vi "PlayinwithRIGOL.vi"() -> ()   [LabVIEW 2009]
panel:
  in  "Wait Duration (us)":dbl
  in  "Pulse Duration (us)":dbl
  in  "Ncycles":u16
  in  "Frequency (MHz)":dbl
  in  "Amplitude (Vpp)":dbl
  in  "Phase (degrees 0-360)":dbl
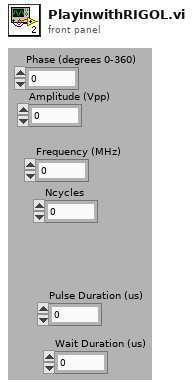
[diagram p1: front panel]
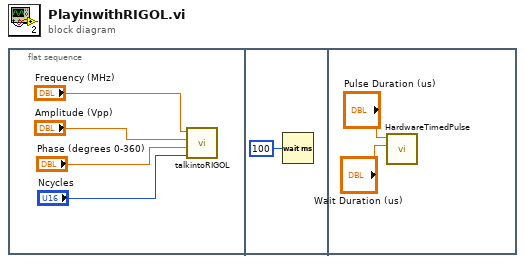
[diagram p0: block diagram]
diagram:
  n1 = flat-sequence {
    frame #0 {
      n2 = call "talkintoRIGOL.vi"("Ncycles"="Ncycles", "Phase (degrees 0-360)"="Phase (degrees 0-360)", "Amplitude (Vpp)"="Amplitude (Vpp)", "Frequency (MHz)"="Frequency (MHz)") -> ()  [unwired: 8 in]
    }
    frame #1 {
      n3 = Wait (ms)(milliseconds to wait=u32 100) -> ()  [unwired: 1 out]
    }
    frame #2 {
      n4 = call "HardwareTimedPulse.vi"("Wait Duration (us)"="Wait Duration (us)", "Pulse Duration (us)"="Pulse Duration (us)") -> ()  [unwired: 10 in]
    }
  }
